vi "AdvFilter-Get Spectrum.vi"(0 "Filter in":T1 {"Stages"."IIR Filter"."Forward Coefficients" format="%.4f"; "Stages"."IIR Filter"."Reverse Coefficients" format="%.4f"}, 5 "Sampling Rate (Hz)":dbl, 7 "Npts":i32, 11 "error in (no error)":errorcluster) -> (4 "Filter out":T1 {"Stages"."IIR Filter"."Forward Coefficients" format="%.4f"; "Stages"."IIR Filter"."Reverse Coefficients" format="%.4f"}, 8 "spectrum":cdb[](array[numeric]), 15 "error out":errorcluster)   [LabVIEW 2020]
uses:
  Controls/Advanced Filter XCtl/Filter Data.ctl
  Filter-Bandwidth Units.ctl
  <vilib>/Analysis/1siggen.llb/Ramp Pattern by Samples.vi
  <vilib>/Analysis/3filter.llb/IIR Cascade Filter with I.C. (DBL).vi
  <vilib>/Analysis/2dsp.llb/Real FFT.vi
  Utility VIs/Math VIs/Linear to dB (array).vi
  <vilib>/Analysis/NI_AALBase.lvlib
  <vilib>/Analysis/NI_AALPro.lvlib
  Controls/Advanced Filter XCtl/Advanced Filter XCtl.xctl
panel:
  out "Magnitude":dbl[](graph)
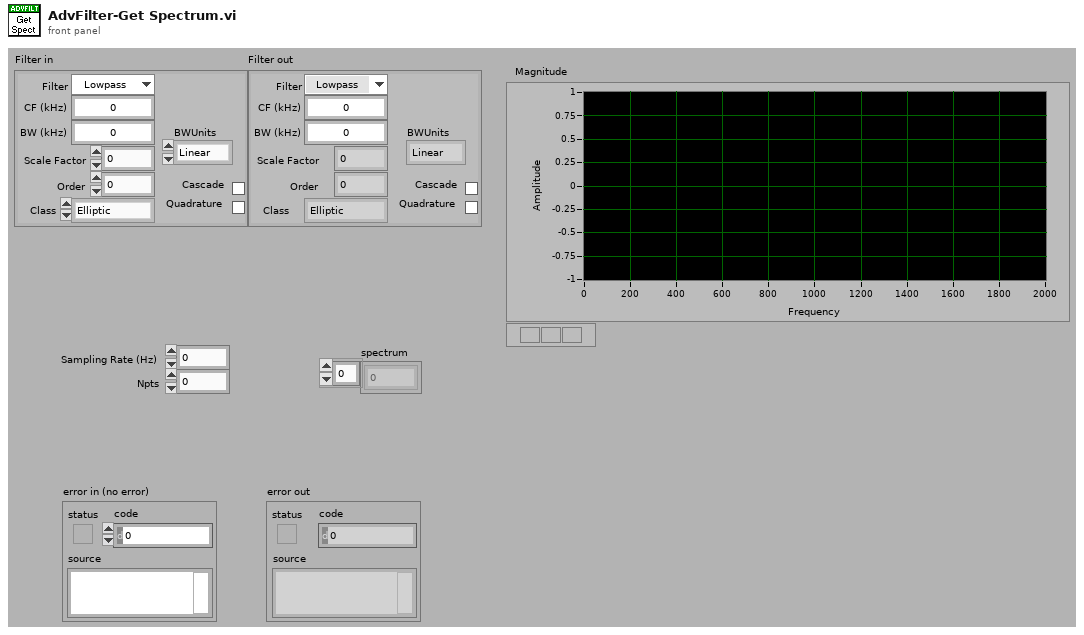
[diagram p1: front panel]
types:
  T1 = typedef "Advanced Filter XCtl.xctl/Filter Data.ctl" = cluster{"Type":enum16{"Lowpass", "Highpass", "Bandpass", "Bandstop", "OFF"}, "CF (kHz)":dbl, "BW (kHz)":dbl, "Cascade":bool, "Quadrature":bool, "Scale Factor":dbl, "Stages":cluster{"IIR Filter":cluster{"filter structure":enum32{"IIR 2nd Order", "IIR 4th Order"}, "Reverse Coefficients":dbl[], "Forward Coefficients":dbl[]}, "State":dbl[]}[], "Class":enum16{"Elliptic", "Butterworth"}, "Order":i32, "BWUnits":T2}
  T2 = typedef "Filter-Bandwidth Units.ctl" = enum16{"Linear", "Octaves", "Min-Max"}
  T3 = enum16{"Lowpass", "Highpass", "Bandpass", "Bandstop", "OFF"}
  T4 = cluster{"IIR Filter":cluster{"filter structure":enum32{"IIR 2nd Order", "IIR 4th Order"}, "Reverse Coefficients":dbl[], "Forward Coefficients":dbl[]}, "State":dbl[]}[]
  T5 = cluster{"IIR Filter":cluster{"filter structure":enum32{"IIR 2nd Order", "IIR 4th Order"}, "Reverse Coefficients":dbl[], "Forward Coefficients":dbl[]}, "State":dbl[]}
  T6 = cluster{"filter structure":enum32{"IIR 2nd Order", "IIR 4th Order"}, "Reverse Coefficients":dbl[], "Forward Coefficients":dbl[]}
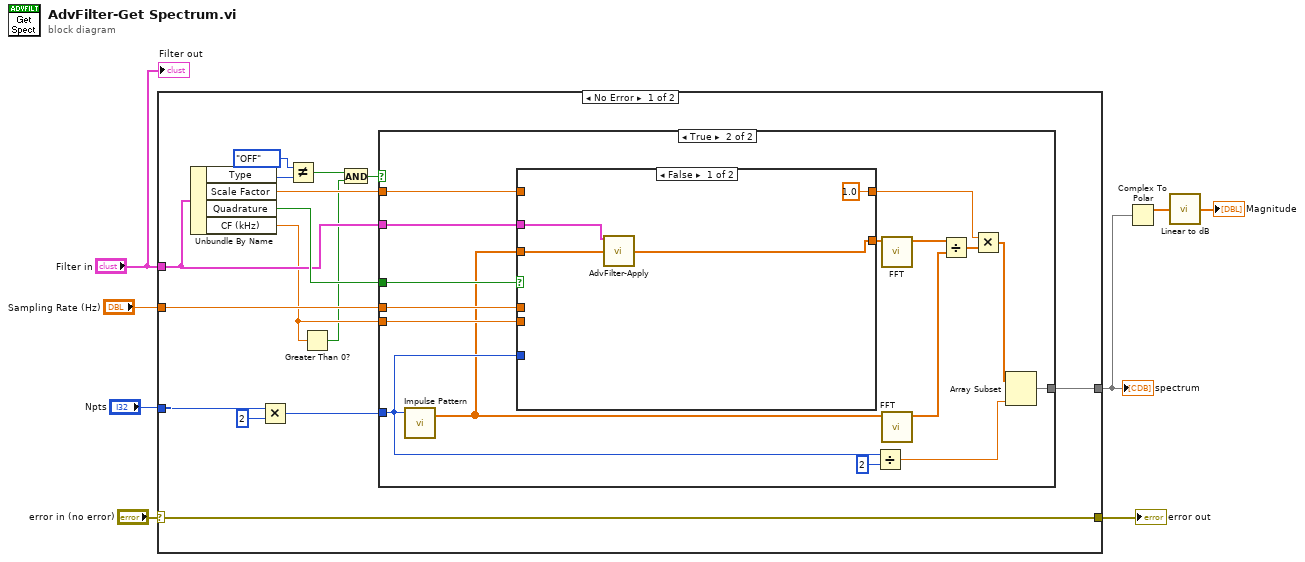
[diagram p0: block diagram]
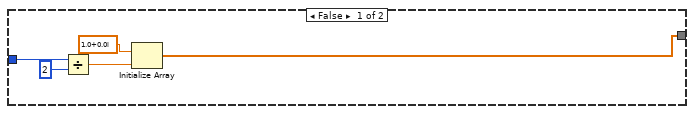
[diagram p2: hidden frame]
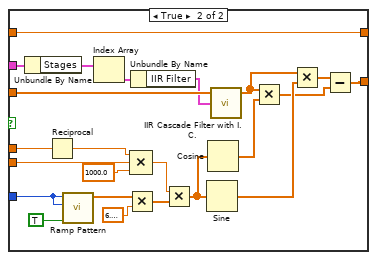
[diagram p3: hidden frame]
diagram:
  n1 = case shown="No Error" "error in (no error)" {
    selector: "error in (no error)" -> [w22 w72]
    tunnel: "Filter in" -> [w12 _]
    tunnel: "Npts" -> [w17 _]
    tunnel: [w23 _] -> w5
    tunnel: [w22 w72] -> w6
    tunnel: "Sampling Rate (Hz)" -> [w16 _]
    frame No Error {
      n2 = Unbundle By Name(w12) -> ("Type"=w15:T3, "Scale Factor"=w21:dbl, "Quadrature"=w18:bool, "CF (kHz)"=w10:dbl)
      n3 = Multiply(x=w17, y=2) -> (x*y=w20:i32)
      n4 = Not Equal?(x=T3."OFF", y=w15) -> (x != y?=w13:bool)
      n5 = Greater Than 0?(x=w10) -> (x > 0?=w9:bool)
      n6 = And(x=w13, y=w9) -> (x .and. y?=w11:bool)
      n7 = case shown="True" w11 {
        tunnel: w20 -> [w27 w33]
        tunnel: [w24 w39] -> w23
        tunnel: w21 -> [_ w29]
        tunnel: w18 -> [_ w36]
        tunnel: w10 -> [_ w35]
        tunnel: w16 -> [_ w34]
        tunnel: w12 -> [_ w31]
        frame False {
          n8 = Divide(x=w27, y=2) -> (x/y=w26:dbl)
          n9 = Initialize Array(cdb 1.0+0.0i ("element"), w26) -> (w24:cdb[])
        }
        frame True {
          n10 = call <vilib>:"Impulse Pattern.vi"("samples"=w33) -> ("Impulse Pattern"=w32:dbl[])  [unwired: 2 in, 1 out]
          n11 = case shown="False" w36 {
            tunnel: w32 -> [w48 w52]
            tunnel: [w46 w60] -> w37
            tunnel: w35 -> [_ w59]
            tunnel: w33 -> [_ w58]
            tunnel: w34 -> [_ w57]
            tunnel: w31 -> [w47 w55]
            tunnel: [1.0 ("Scale Factor") w49] -> w30
            tunnel: w29 -> [_ w49]
            frame False {
              n12 = call "AdvFilter-Apply.vi"("Filter"=w47, "X"=w48) -> ("Filtered X"=w46:dbl[])  [unwired: 11 in, 2 out]
            }
            frame True {
              n13 = Unbundle By Name(w55) -> ("Stages"=w54:T4)
              n14 = Reciprocal(x=w57) -> (1/x=w56:dbl)
              n15 = call-poly <vilib>:"Ramp Pattern.vi"("exclude end?"=TRUE, "end"=w58, "samples"=w58) -> ("Ramp Pattern"=w70:dbl[])  [unwired: 7 in, 1 out]
              n16 = Index Array(array=w54) -> (element=w53:T5)  [unwired: 1 in]
              n17 = Multiply(x=w70, y=6.283185307179586) -> (x*y=w69:dbl[])
              n18 = Compound Arithmetic op=MULTIPLY(w56, w59, 1000.0 ("y")) -> (w62:dbl)
              n19 = Unbundle By Name(w53) -> ("IIR Filter"=w51:T6)
              n20 = Multiply(x=w62, y=w69) -> (x*y=w67:dbl[])
              n21 = Sine(x=w67) -> (sin(x)=w68:dbl[])
              n22 = Cosine(x=w67) -> (cos(x)=w66:dbl[])
              n23 = call-poly <vilib>:"IIR Cascade Filter with I.C..vi"("IIR Filter Cluster"=w51, "X"=w52) -> ("Filtered X"=w50:dbl[])  [unwired: 1 in, 2 out]
              n24 = Multiply(x=w50, y=w66) -> (x*y=w64:dbl[])
              n25 = Multiply(x=w50, y=w68) -> (x*y=w65:dbl[])
              n26 = Subtract(x=w65, y=w64) -> (x-y=w60:dbl[])
            }
          }
          n27 = Divide(x=w33, y=2) -> (x/y=w40:dbl)
          n28 = call-poly <vilib>:"FFT.vi"("X"=w37) -> ("FFT {X}"=w44:cdb[])  [unwired: 9 in, 1 out]
          n29 = call-poly <vilib>:"FFT.vi"("X"=w32) -> ("FFT {X}"=w43:cdb[])  [unwired: 9 in, 1 out]
          n30 = Divide(x=w44, y=w43) -> (x/y=w42:cdb[])
          n31 = Multiply(x=w30, y=w42) -> (x*y=w38:cdb[])
          n32 = Array Subset(array=w38, length=w40) -> (w39:cdb[])  [unwired: 1 in]
        }
      }
    }
    frame Error {
    }
  }
  "error out" <- w6
  "spectrum" <- w5
  n33 = Complex To Polar(r * e^(i*theta)=w5) -> (r=w4:dbl[])  [unwired: 1 out]
  n34 = call-poly "Linear to dB.vi"("linear"=w4) -> ("dB"=→"Magnitude":dbl[])
  "Filter out" <- "Filter in"
